vi "Choose Random Command.vi"(1 "Array":string[](array[string])) -> (0 "String":string)   [LabVIEW 2019, in "RemoteControl.lvclass"]
uses:
  <vilib>/numeric/Random Number (Range) U64.vi
  <vilib>/numeric/sub_Random U32.vi
  RemoteControl.lvclass
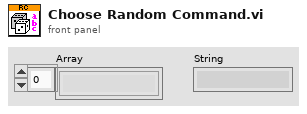
[diagram p1: front panel]
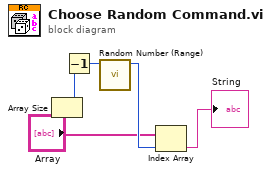
[diagram p0: block diagram]
diagram:
  n1 = Array Size(array="Array") -> (size(s)=w1:i32)
  n2 = Decrement(x=w1) -> (x-1=w3:i32)
  n3 = call-poly <vilib>:"Random Number (Range).vi"("upper bound (100)"=w3) -> ("number"=w4:u64)  [unwired: 10 in]
  n4 = Index Array(array="Array", index=w4) -> (element=→"String":string)
